vi "tag_lens_trigger.vi"(0 "previous DIO value":bool) -> (1 "DIO to shift registar":bool, 2 "trigger out":bool)   [LabVIEW 2010]
uses:
  <vilib>/eio/EIONode/EIONode.xnode
  <vilib>/rvi/eio/nirviEIOImplementation/nirviEIOImplementation.xnode
  <vilib>/rvi/eio/common/nirviEmuClasses.ctl
  <vilib>/rvi/eio/common/nirviEmuTemplateMethod_noerrors.vi
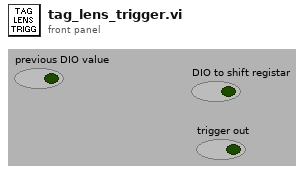
[diagram p1: front panel]
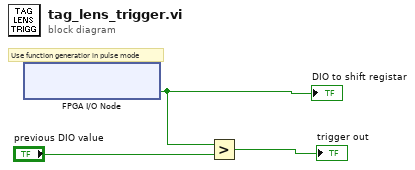
[diagram p0: block diagram]
diagram:
  # "Use function generatior in pulse mode"
  n1 = xnode "FPGA I/O Node"() -> ("Connector0/DIO6"=w3:bool)  [unwired: 1 in, 1 out]
  "DIO to shift registar" <- w3
  n2 = Greater?(x=w3, y="previous DIO value") -> (0:→"trigger out":bool)
